vi "mean_and_std_plot.vi"() -> ()   [LabVIEW 2021]
uses:
  <vilib>/Analysis/NI_AALBase.lvlib
panel:
  out "XY Graph":cluster{i32[], "Y":dbl[]}[](graph)
  out "STDEV":dbl
  out "Mean":dbl
  out "x-y":dbl[](array[numeric])
  out "X":dbl[](array[numeric])
  in  "Y":dbl[](array[numeric])
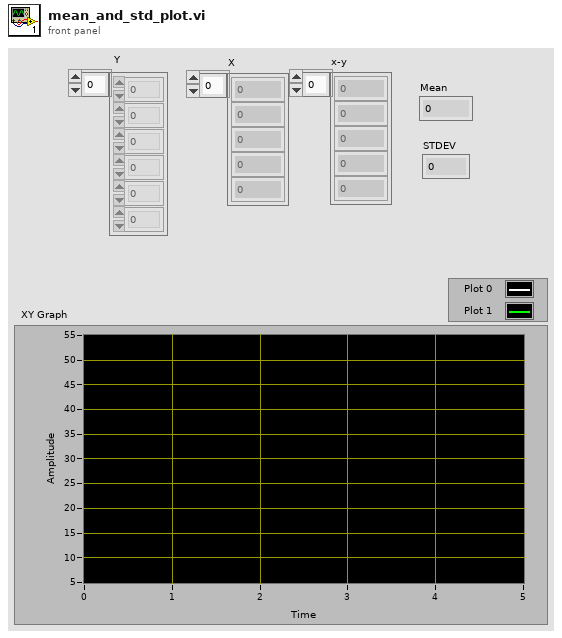
[diagram p1: front panel]
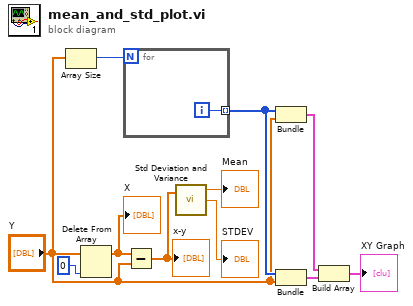
[diagram p0: block diagram]
diagram:
  n1 = Array Size(array="Y") -> (size(s)=w7:i32)
  n2 = Delete From Array(array="Y", index=0) -> (array with subset deleted=w10:dbl[])  [unwired: 1 in, 1 out]
  "X" <- w10
  n3 = for {
    N: w7 -> [_]
    tunnel: [w12] -> w5 mode=indexing
    i -> [w12]
  }
  n4 = Subtract(x=w10, y="Y") -> (x-y=w6:dbl[])
  "x-y" <- w6
  n5 = call <vilib>:"Std Deviation and Variance.vi"("X"=w6) -> ("mean"=→"Mean":dbl, "standard deviation"=→"STDEV":dbl)  [unwired: 1 in, 1 out]
  n6 = Bundle(w5, "Y"="Y") -> (w3:cluster{i32[], "Y":dbl[]})  [unwired: 1 in]
  n7 = Bundle(w5, "Y"="Y") -> (w2:cluster{i32[], "Y":dbl[]})  [unwired: 1 in]
  n8 = Build Array(w3, w2) -> (→"XY Graph":cluster{i32[], "Y":dbl[]}[])
